vi "sub_saveScreen.vi"(8 "에러 입력(에러 없음)":errorcluster, 9 "파일명":string, 10 "저장경로":path, 11 "VISA 참조 번호 입력":refnum<visa-resource-name>) -> (0 "에러 출력":errorcluster, 3 "VISA 참조 번호 출력":refnum<visa-resource-name>)   [LabVIEW 2020]
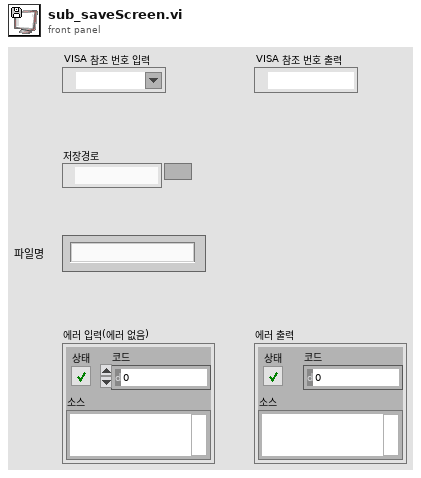
[diagram p1: front panel]
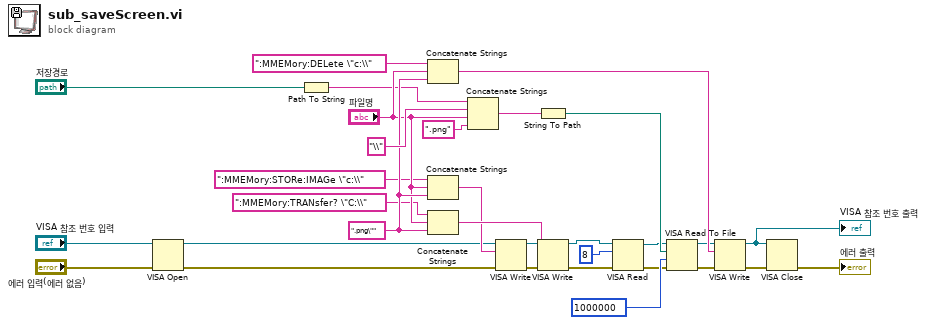
[diagram p0: block diagram]
diagram:
  w27 = ".png\"" ("문자열")
  n1 = VISA Open(error in (no error)="에러 입력(에러 없음)", VISA resource name="VISA 참조 번호 입력") -> (VISA resource name=w2:refnum<visa-resource-name>, error out=w3:errorcluster)  [unwired: 3 in]
  n2 = Path To String(path="저장경로") -> (string=w17:string)
  n3 = Concatenate Strings(":MMEMory:DELete \"c:\\" ("버퍼 쓰기"), "파일명", w27) -> (w24:string)
  n4 = Concatenate Strings(":MMEMory:STORe:IMAGe \"c:\\" ("버퍼 쓰기"), "파일명", w27) -> (w11:string)
  n5 = Concatenate Strings(":MMEMory:TRANsfer? \"C:\\" ("버퍼 쓰기"), "파일명", w27) -> (w13:string)
  n6 = Concatenate Strings(w17, "\\" ("문자열"), "파일명", ".png" ("문자열")) -> (w18:string)
  n7 = VISA Write(VISA resource name=w2, write buffer=w11, error in (no error)=w3) -> (VISA resource name out=w4:refnum<visa-resource-name>, error out=w5:errorcluster)  [unwired: 1 out]
  n8 = String To Path(string=w18) -> (path=w19:path)
  n9 = VISA Write(VISA resource name=w4, write buffer=w13, error in (no error)=w5) -> (VISA resource name out=w6:refnum<visa-resource-name>, error out=w7:errorcluster)  [unwired: 1 out]
  n10 = VISA Read(VISA resource name=w6, byte count=u32 8 ("바이트 카운트"), error in (no error)=w7) -> (VISA resource name out=w15:refnum<visa-resource-name>, error out=w16:errorcluster)  [unwired: 2 out]
  n11 = VISA Read To File(8:w16, 9:u32 1000000 ("바이트 카운트"), 10:w19, 11:w15) -> (0:w22:errorcluster, 3:w21:refnum<visa-resource-name>)  [unwired: 1 out]
  n12 = VISA Write(VISA resource name=w21, write buffer=w24, error in (no error)=w22) -> (VISA resource name out=w31:refnum<visa-resource-name>, error out=w25:errorcluster)  [unwired: 1 out]
  "VISA 참조 번호 출력" <- w31
  n13 = VISA Close(VISA resource name=w31, error in (no error)=w25) -> (error out=→"에러 출력":errorcluster)
